vi "Read Waveform Measurement.vi"(8 "error in (no error)":errorcluster, 9 "Measurement Function (0: Voltage Vpp)":u16(ring) items=["Voltage Vpp", "Voltage Max", "Voltage Min", "Amplitude", "Voltage TOP", "Voltage Base", "Voltage Average", "Voltage RMS", "Overshoot", "Preshoot", "Frequency", "Rise Time", "Fall Time", "Period", "Positive Width", "Negative Width", "Positive Duty", "Negative Duty"], 10 "Source (0: Channel 1)":u16(ring) items=["Channel 1", "Channel 2", "Channel 3", "Channel 4"], 11 "VISA resource name":refnum<visa-resource-name>) -> (0 "error out":errorcluster, 2 "Measured Value":dbl, 3 "VISA resource name out":refnum<visa-resource-name>)   [LabVIEW 2015, in "RIGOL DS1000 Series.lvlib"]
doc: "Read waveform measurement from oscilloscope."
uses:
  RIGOL DS1000 Series.lvlib
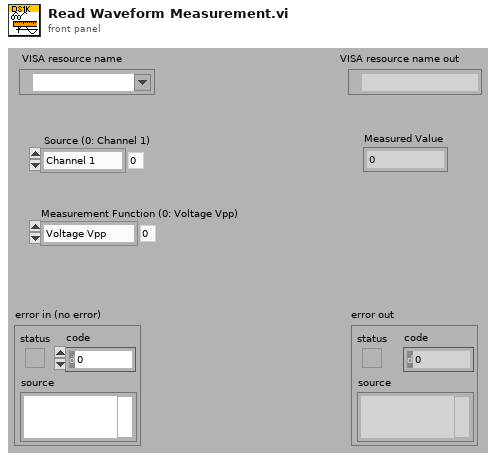
[diagram p1: front panel]
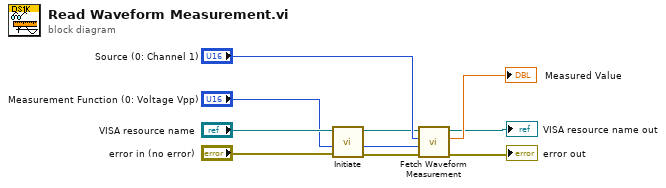
[diagram p0: block diagram]
diagram:
  n1 = call "Initiate.vi"("error in (no error)"="error in (no error)", "VISA resource name"="VISA resource name") -> ("error out"=w4:errorcluster, "VISA resource name out"=w5:refnum<visa-resource-name>)  [unwired: 8 out]
  n2 = call "Fetch Waveform Measurement.vi"("error in (no error)"=w4, "Measurement Function (0: Voltage Vpp)"="Measurement Function (0: Voltage Vpp)", "Source (0: Channel 1)"="Source (0: Channel 1)", "VISA resource name"=w5) -> ("error out"=→"error out":errorcluster, "Measured Value"=→"Measured Value":dbl, "VISA resource name out"=→"VISA resource name out":refnum<visa-resource-name>)  [unwired: 5 out]
